vi "Message test FGV.vi"(6 "Enum":enum16{"Add", "Reset"}(ring), 11 "String":string) -> (3 "out":string[](array[string]))   [LabVIEW 2016]
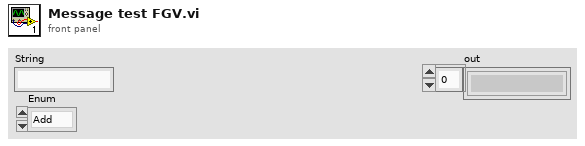
[diagram p1: front panel]
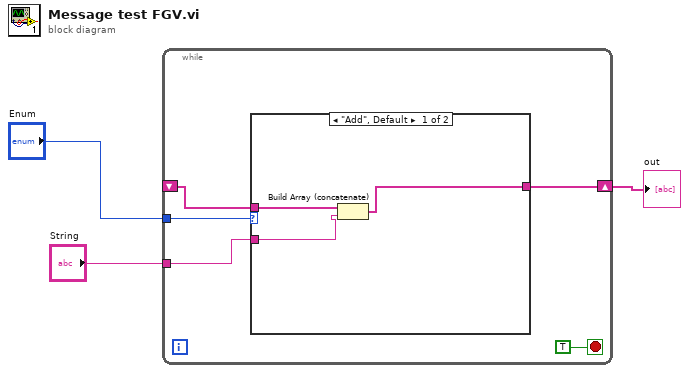
[diagram p0: block diagram]
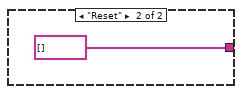
[diagram p2: hidden frame]
diagram:
  n1 = while {
    tunnel: "String" -> [w8]
    tunnel: "Enum" -> [w7]
    shift-right: [w6] -> w1
    shift-left: _ -> [w5]
    stop <- TRUE stop-if-true
    n2 = case shown="\"Add\", Default" w7 {
      tunnel: w8 -> [w11 _]
      tunnel: [w10 string[] [] ("appended array")] -> w6
      tunnel: w5 -> [w9 _]
      frame "Add", Default {
        n3 = Build Array (concatenate)(w9, w11) -> (w10:string[])
      }
      frame "Reset" {
      }
    }
  }
  "out" <- w1
